vi "Checksum.vi"(1 "Sum of bytes":u8) -> (0 "Checksum String":string)   [LabVIEW 2016, in "Dynamixel Motor.lvlib"]
doc: "Computes the checksum for the serial message."
uses:
  Dynamixel Motor.lvlib
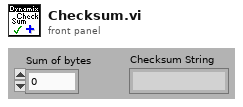
[diagram p1: front panel]
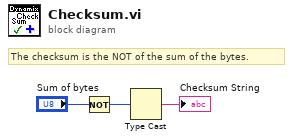
[diagram p0: block diagram]
diagram:
  # "The checksum is the NOT of the sum of the bytes."
  n1 = Not(x="Sum of bytes") -> (.not. x?=w2:u8)
  n2 = Type Cast(x=w2) -> (*(type *) &x=→"Checksum String":string)  [unwired: 1 in]
